vi "main.vi"() -> ()   [LabVIEW 2023] (continued)
 0CF102A7   00000004    8        30\t75\tE0\t2E\t80\tFF\tFF\tFD\r\n       463  0CF101A7   00000004    8        68\t00\t97\tCC\t00\t15\t39\t31\r\n       512  1FFFFFFF   00000004    8        00\t20\tFF\tFF\tFF\tFF\tFF\tFF\r\n       503  0CF102A7   00000004    8        30\t75\tE0\t2E\t80\tFF\tFF\tFD\r\n       503  0CF101A7   00000004    8        68\t00\t97\tCC\t00\t15\t39\t33\r\n       502  1FFFFFFF   00000004    8        00\t20\tFF\tFF\tFF\tFF\tFF\tFF\r\n       493  18F106A7   00000004    8        00\tF7\tFF\tFF\tFF\tFF\tFF\t7A\r\n       492  1FFFFFFF   00000004    8        00\t00\tFF\tFF\tFF\tFF\tFF\tFF\r\n       483  0CF102A7   00000004    8        30\t75\tE0\t2E\t80\tFF\tFF\tFD\r\n       483  0CF101A7   00000004    8        68\t00\t97\tCC\t00\t15\t39\t32\r\n       482  1FFFFFFF   00000004    8        00\t20\tFF\tFF\tFF\tFF\tFF\tFF\r\n       472  1FFFFFFF   00000004    8        00\t20\tFF\tFF\tFF\tFF\tFF\tFF\r\n       463  0CF102A7   00000004    8        30\t75\tE0\t2E\t80\tFF\tFF\tFD\r\n       522  1FFFFFFF   00000004    8        00\t20\tFF\tFF\tFF\tFF\tFF\tFF\r\n       512  1FFFFFFF   00000004    8        00\t20\tFF\tFF\tFF\tFF\tFF\tFF\r\n       503  0CF102A7   00000004    8        30\t75\tE0\t2E\t80\tFF\tFF\tFD\r\n       503  0CF101A7   00000004    8        68\t00\t97\tCC\t00\t15\t39\t33\r\n       502  1FFFFFFF   00000004    8        00\t20\tFF\tFF\tFF\tFF\tFF\tFF\r\n       493  18F106A7   00000004    8        00\tF7\tFF\tFF\tFF\tFF\tFF\t7A\r\n       492  1FFFFFFF   00000004    8        00\t00\tFF\tFF\tFF\tFF\tFF\tFF\r\n       483  0CF102A7   00000004    8        30\t75\tE0\t2E\t80\tFF\tFF\tFD\r\n       483  0CF101A7   00000004    8        68\t00\t97\tCC\t00\t15\t39\t32\r\n       482  1FFFFFFF   00000004    8        00\t20\tFF\tFF\tFF\tFF\tFF\tFF\r\n       472  1FFFFFFF   00000004    8        00\t20\tFF\tFF\tFF\tFF\tFF\tFF\r\n       523  0CF101A7   00000004    8        68\t00\t97\tCC\t00\t15\t39\t34\r\n       522  1FFFFFFF   00000004    8        00\t20\tFF\tFF\tFF\tFF\tFF\tFF\r\n       512  1FFFFFFF   00000004    8        00\t20\tFF\tFF\tFF\tFF\tFF\tFF\r\n       503  0CF102A7   00000004    8        30\t75\tE0\t2E\t80\tFF\tFF\tFD\r\n       503  0CF101A7   00000004    8        68\t00\t97\tCC\t00\t15\t39\t33\r\n       502  1FFFFFFF   00000004    8        00\t20\tFF\tFF\tFF\tFF\tFF\tFF\r\n       493  18F106A7   00000004    8        00\tF7\tFF\tFF\tFF\tFF\tFF\t7A\r\n       492  1FFFFFFF   00000004    8        00\t00\tFF\tFF\tFF\tFF\tFF\tFF\r\n       483  0CF102A7   00000004    8        30\t75\tE0\t2E\t80\tFF\tFF\tFD\r\n       483  0CF101A7   00000004    8        68\t00\t97\tCC\t00\t15\t39\t32\r\n       482  1FFFFFFF   00000004    8        00\t20\tFF\tFF\tFF\tFF\tFF\tFF\r\n       523  0CF102A7   00000004    8        30\t75\tE0\t2E\t80\tFF\tFF\tFD\r\n       523  0CF101A7   00000004    8        68\t00\t97\tCC\t00\t15\t39\t34\r\n       522  1FFFFFFF   00000004    8        00\t20\tFF\tFF\tFF\tFF\tFF\tFF\r\n       512  1FFFFFFF   00000004    8        00\t20\tFF\tFF\tFF\tFF\tFF\tFF\r\n       503  0CF102A7   00000004    8        30\t75\tE0\t2E\t80\tFF\tFF\tFD\r\n       503  0CF101A7   00000004    8        68\t00\t97\tCC\t00\t15\t39\t33\r\n       502  1FFFFFFF   00000004    8        00\t20\tFF\tFF\tFF\tFF\tFF\tFF\r\n       493  18F106A7   00000004    8        00\tF7\tFF\tFF\tFF\tFF\tFF\t7A\r\n       492  1FFFFFFF   00000004    8        00\t00\tFF\tFF\tFF\tFF\tFF\tFF\r\n       483  0CF102A7   00000004    8        30\t75\tE0\t2E\t80\tFF\tFF\tFD\r\n       483  0CF101A7   00000004    8        68\t00\t97\tCC\t00\t15\t39\t32\r\n       532  1FFFFFFF   00000004    8        00\t20\tFF\tFF\tFF\tFF\tFF\tFF\r\n       523  0CF102A7   00000004    8        30\t75\tE0\t2E\t80\tFF\tFF\tFD\r\n       523  0CF101A7   00000004    8        68\t00\t97\tCC\t00\t15\t39\t34\r\n       522  1FFFFFFF   00000004    8        00\t20\tFF\tFF\tFF\tFF\tFF\tFF\r\n       512  1FFFFFFF   00000004    8        00\t20\tFF\tFF\tFF\tFF\tFF\tFF\r\n       503  0CF102A7   00000004    8        30\t75\tE0\t2E\t80\tFF\tFF\tFD\r\n       503  0CF101A7   00000004    8        68\t00\t97\tCC\t00\t15\t39\t33\r\n       502  1FFFFFFF   00000004    8        00\t20\tFF\tFF\tFF\tFF\tFF\tFF\r\n       493  18F106A7   00000004    8        00\tF7\tFF\tFF\tFF\tFF\tFF\t7A\r\n       492  1FFFFFFF   00000004    8        00\t00\tFF\tFF\tFF\tFF\tFF\tFF\r\n       483  0CF102A7   00000004    8        30\t75\tE0\t2E\t80\tFF\tFF\tFD\r\n       541  18F11FF0   00000004    8        FF\t3F\t90\t68\t88\t1B\t10\tDC\r\n       532  1FFFFFFF   00000004    8        00\t20\tFF\tFF\tFF\tFF\tFF\tFF\r\n       523  0CF102A7   00000004    8        30\t75\tE0\t2E\t80\tFF\tFF\tFD\r\n       523  0CF101A7   00000004    8        68\t00\t97\tCC\t00\t15\t39\t34\r\n       522  1FFFFFFF   00000004    8        00\t20\tFF\tFF\tFF\tFF\tFF\tFF\r\n       512  1FFFFFFF   00000004    8        00\t20\tFF\tFF\tFF\tFF\tFF\tFF\r\n       503  0CF102A7   00000004    8        30\t75\tE0\t2E\t80\tFF\tFF\tFD\r\n       503  0CF101A7   00000004    8        68\t00\t97\tCC\t00\t15\t39\t33\r\n       502  1FFFFFFF   00000004    8        00\t20\tFF\tFF\tFF\tFF\tFF\tFF\r\n       493  18F106A7   00000004    8        00\tF7\tFF\tFF\tFF\tFF\tFF\t7A\r\n       492  1FFFFFFF   00000004    8        00\t00\tFF\tFF\tFF\tFF\tFF\tFF\r\n       542  18F120F0   00000004    8        2B\t75\t60\tB1\tB0\t01\tFF\tFF\r\n       541  18F11FF0   00000004    8        FF\t3F\t90\t68\t88\t1B\t10\tDC\r\n       532  1FFFFFFF   00000004    8        00\t20\tFF\tFF\tFF\tFF\tFF\tFF\r\n       523  0CF102A7   00000004    8        30\t75\tE0\t2E\t80\tFF\tFF\tFD\r\n       523  0CF101A7   00000004    8        68\t00\t97\tCC\t00\t15\t39\t34\r\n       522  1FFFFFFF   00000004    8        00\t20\tFF\tFF\tFF\tFF\tFF\tFF\r\n       512  1FFFFFFF   00000004    8        00\t20\tFF\tFF\tFF\tFF\tFF\tFF\r\n       503  0CF102A7   00000004    8        30\t75\tE0\t2E\t80\tFF\tFF\tFD\r\n       503  0CF101A7   00000004    8        68\t00\t97\tCC\t00\t15\t39\t33\r\n       502  1FFFFFFF   00000004    8        00\t20\tFF\tFF\tFF\tFF\tFF\tFF\r\n       493  18F106A7   00000004    8        00\tF7\tFF\tFF\tFF\tFF\tFF\t7A\r\n       543  0CF101A7   00000004    8        68\t00\t97\tCC\t00\t15\t39\t35\r\n       542  18F120F0   00000004    8        2B\t75\t60\tB1\tB0\t01\tFF\tFF\r\n       541  18F11FF0   00000004    8        FF\t3F\t90\t68\t88\t1B\t10\tDC\r\n       532  1FFFFFFF   00000004    8        00\t20\tFF\tFF\tFF\tFF\tFF\tFF\r\n       523  0CF102A7   00000004    8        30\t75\tE0\t2E\t80\tFF\tFF\tFD\r\n       523  0CF101A7   00000004    8        68\t00\t97\tCC\t00\t15\t39\t34\r\n       522  1FFFFFFF   00000004    8        00\t20\tFF\tFF\tFF\tFF\tFF\tFF\r\n       512  1FFFFFFF   00000004    8        00\t20\tFF\tFF\tFF\tFF\tFF\tFF\r\n       503  0CF102A7   00000004    8        30\t75\tE0\t2E\t80\tFF\tFF\tFD\r\n       503  0CF101A7   00000004    8        68\t00\t97\tCC\t00\t15\t39\t33\r\n       502  1FFFFFFF   00000004    8        00\t20\tFF\tFF\tFF\tFF\tFF\tFF\r\n       543  0C3C4D4A   00000004    8        BE\tFF\tFF\t7F\t18\tFF\tFF\t3D\r\n       543  0CF101A7   00000004    8        68\t00\t97\tCC\t00\t15\t39\t35\r\n       542  18F120F0   00000004    8        2B\t75\t60\tB1\tB0\t01\tFF\tFF\r\n       541  18F11FF0   00000004    8        FF\t3F\t90\t68\t88\t1B\t10\tDC\r\n       532  1FFFFFFF   00000004    8        00\t20\tFF\tFF\tFF\tFF\tFF\tFF\r\n       523  0CF102A7   00000004    8        30\t75\tE0\t2E\t80\tFF\tFF\tFD\r\n       523  0CF101A7   00000004    8        68\t00\t97\tCC\t00\t15\t39\t34\r\n       522  1FFFFFFF   00000004    8        00\t20\tFF\tFF\tFF\tFF\tFF\tFF\r\n       512  1FFFFFFF   00000004    8        00\t20\tFF\tFF\tFF\tFF\tFF\tFF\r\n       503  0CF102A7   00000004    8        30\t75\tE0\t2E\t80\tFF\tFF\tFD\r\n       503  0CF101A7   00000004    8        68\t00\t97\tCC\t00\t15\t39\t33\r\n       544  0CF102A7   00000004    8        30\t75\tE0\t2E\t80\tFF\tFF\tFD\r\n       543  0C3C4D4A   00000004    8        BE\tFF\tFF\t7F\t18\tFF\tFF\t3D\r\n       543  0CF101A7   00000004    8        68\t00\t97\tCC\t00\t15\t39\t35\r\n       542  18F120F0   00000004    8        2B\t75\t60\tB1\tB0\t01\tFF\tFF\r\n       541  18F11FF0   00000004    8        FF\t3F\t90\t68\t88\t1B\t10\tDC\r\n       532  1FFFFFFF   00000004    8        00\t20\tFF\tFF\tFF\tFF\tFF\tFF\r\n       523  0CF102A7   00000004    8        30\t75\tE0\t2E\t80\tFF\tFF\tFD\r\n       523  0CF101A7   00000004    8        68\t00\t97\tCC\t00\t15\t39\t34\r\n       522  1FFFFFFF   00000004    8        00\t20\tFF\tFF\tFF\tFF\tFF\tFF\r\n       512  1FFFFFFF   00000004    8        00\t20\tFF\tFF\tFF\tFF\tFF\tFF\r\n       503  0CF102A7   00000004    8        30\t75\tE0\t2E\t80\tFF\tFF\tFD\r\n       544  0CF103A7   00000004    8        17\t1F\t08\t60\tB1\t1F\t08\t3D\r\n       544  0CF102A7   00000004    8        30\t75\tE0\t2E\t80\tFF\tFF\tFD\r\n       543  0C3C4D4A   00000004    8        BE\tFF\tFF\t7F\t18\tFF\tFF\t3D\r\n       543  0CF101A7   00000004    8        68\t00\t97\tCC\t00\t15\t39\t35\r\n       542  18F120F0   00000004    8        2B\t75\t60\tB1\tB0\t01\tFF\tFF\r\n       541  18F11FF0   00000004    8        FF\t3F\t90\t68\t88\t1B\t10\tDC\r\n       532  1FFFFFFF   00000004    8        00\t20\tFF\tFF\tFF\tFF\tFF\tFF\r\n       523  0CF102A7   00000004    8        30\t75\tE0\t2E\t80\tFF\tFF\tFD\r\n       523  0CF101A7   00000004    8        68\t00\t97\tCC\t00\t15\t39\t34\r\n       522  1FFFFFFF   00000004    8        00\t20\tFF\tFF\tFF\tFF\tFF\tFF\r\n       512  1FFFFFFF   00000004    8        00\t20\tFF\tFF\tFF\tFF\tFF\tFF\r\n       545  0CF104A7   00000004    8        F0\t60\t22\tFC\tFF\tFF\tFF\t3D\r\n       544  0CF103A7   00000004    8        17\t1F\t08\t60\tB1\t1F\t08\t3D\r\n       544  0CF102A7   00000004    8        30\t75\tE0\t2E\t80\tFF\tFF\tFD\r\n       543  0C3C4D4A   00000004    8        BE\tFF\tFF\t7F\t18\tFF\tFF\t3D\r\n       543  0CF101A7   00000004    8        68\t00\t97\tCC\t00\t15\t39\t35\r\n       542  18F120F0   00000004    8        2B\t75\t60\tB1\tB0\t01\tFF\tFF\r\n       541  18F11FF0   00000004    8        FF\t3F\t90\t68\t88\t1B\t10\tDC\r\n       532  1FFFFFFF   00000004    8        00\t20\tFF\tFF\tFF\tFF\tFF\tFF\r\n       523  0CF102A7   00000004    8        30\t75\tE0\t2E\t80\tFF\tFF\tFD\r\n       523  0CF101A7   00000004    8        68\t00\t97\tCC\t00\t15\t39\t34\r\n       522  1FFFFFFF   00000004    8        00\t20\tFF\tFF\tFF\tFF\tFF\tFF\r\n       545  18F106A7   00000004    8        00\tF7\tFF\tFF\tFF\tFF\tFF\t7B\r\n       545  0CF104A7   00000004    8        F0\t60\t22\tFC\tFF\tFF\tFF\t3D\r\n       544  0CF103A7   00000004    8        17\t1F\t08\t60\tB1\t1F\t08\t3D\r\n       544  0CF102A7   00000004    8        30\t75\tE0\t2E\t80\tFF\tFF\tFD\r\n       543  0C3C4D4A   00000004    8        BE\tFF\tFF\t7F\t18\tFF\tFF\t3D\r\n       543  0CF101A7   00000004    8        68\t00\t97\tCC\t00\t15\t39\t35\r\n       542  18F120F0   00000004    8        2B\t75\t60\tB1\tB0\t01\tFF\tFF\r\n       541  18F11FF0   00000004    8        FF\t3F\t90\t68\t88\t1B\t10\tDC\r\n       532  1FFFFFFF   00000004    8        00\t20\tFF\tFF\tFF\tFF\tFF\tFF\r\n       523  0CF102A7   00000004    8        30\t75\tE0\t2E\t80\tFF\tFF\tFD\r\n       523  0CF101A7   00000004    8        68\t00\t97\tCC\t00\t15\t39\t34\r\n       546  18F121F0   00000004    8        09\t16\t00\t00\tFF\tFF\tB0\t01\r\n       545  18F106A7   00000004    8        00\tF7\tFF\tFF\tFF\tFF\tFF\t7B\r\n       545  0CF104A7   00000004    8        F0\t60\t22\tFC\tFF\tFF\tFF\t3D\r\n       544  0CF103A7   00000004    8        17\t1F\t08\t60\tB1\t1F\t08\t3D\r\n       544  0CF102A7   00000004    8        30\t75\tE0\t2E\t80\tFF\tFF\tFD\r\n       543  0C3C4D4A   00000004    8        BE\tFF\tFF\t7F\t18\tFF\tFF\t3D\r\n       543  0CF101A7   00000004    8        68\t00\t97\tCC\t00\t15\t39\t35\r\n       542  18F120F0   00000004    8        2B\t75\t60\tB1\tB0\t01\tFF\tFF\r\n       541  18F11FF0   00000004    8        FF\t3F\t90\t68\t88\t1B\t10\tDC\r\n       532  1FFFFFFF   00000004    8        00\t20\tFF\tFF\tFF\tFF\tFF\tFF\r\n       523  0CF102A7   00000004    8        30\t75\tE0\t2E\t80\tFF\tFF\tFD\r\n       547  1FFFFFFF   00000004    8        00\t00\tFF\tFF\tFF\tFF\tFF\tFF\r\n       546  18F121F0   00000004    8        09\t16\t00\t00\tFF\tFF\tB0\t01\r\n       545  18F106A7   00000004    8        00\tF7\tFF\tFF\tFF\tFF\tFF\t7B\r\n       545  0CF104A7   00000004    8        F0\t60\t22\tFC\tFF\tFF\tFF\t3D\r\n       544  0CF103A7   00000004    8        17\t1F\t08\t60\tB1\t1F\t08\t3D\r\n       544  0CF102A7   00000004    8        30\t75\tE0\t2E\t80\tFF\tFF\tFD\r\n       543  0C3C4D4A   00000004    8        BE\tFF\tFF\t7F\t18\tFF\tFF\t3D\r\n       543  0CF101A7   00000004    8        68\t00\t97\tCC\t00\t15\t39\t35\r\n       542  18F120F0   00000004    8        2B\t75\t60\tB1\tB0\t01\tFF\tFF\r\n       541  18F11FF0   00000004    8        FF\t3F\t90\t68\t88\t1B\t10\tDC\r\n       532  1FFFFFFF   00000004    8        00\t20\tFF\tFF\tFF\tFF\tFF\tFF\r\n       552  1FFFFFFF   00000004    8        00\t20\tFF\tFF\tFF\tFF\tFF\tFF\r\n       547  1FFFFFFF   00000004    8        00\t00\tFF\tFF\tFF\tFF\tFF\tFF\r\n       546  18F121F0   00000004    8        09\t16\t00\t00\tFF\tFF\tB0\t01\r\n       545  18F106A7   00000004    8        00\tF7\tFF\tFF\tFF\tFF\tFF\t7B\r\n       545  0CF104A7   00000004    8        F0\t60\t22\tFC\tFF\tFF\tFF\t3D\r\n       544  0CF103A7   00000004    8        17\t1F\t08\t60\tB1\t1F\t08\t3D\r\n       544  0CF102A7   00000004    8        30\t75\tE0\t2E\t80\tFF\tFF\tFD\r\n       543  0C3C4D4A   00000004    8        BE\tFF\tFF\t7F\t18\tFF\tFF\t3D\r\n       543  0CF101A7   00000004    8        68\t00\t97\tCC\t00\t15\t39\t35\r\n       542  18F120F0   00000004    8        2B\t75\t60\tB1\tB0\t01\tFF\tFF\r\n       541  18F11FF0   00000004    8        FF\t3F\t90\t68\t88\t1B\t10\tDC\r\n       562  1FFFFFFF   00000004    8        00\t00\tFF\tFF\tFF\tFF\tFF\tFF\r\n       552  1FFFFFFF   00000004    8        00\t20\tFF\tFF\tFF\tFF\tFF\tFF\r\n       547  1FFFFFFF   00000004    8        00\t00\tFF\tFF\tFF\tFF\tFF\tFF\r\n       546  18F121F0   00000004    8        09\t16\t00\t00\tFF\tFF\tB0\t01\r\n       545  18F106A7   00000004    8        00\tF7\tFF\tFF\tFF\tFF\tFF\t7B\r\n       545  0CF104A7   00000004    8        F0\t60\t22\tFC\tFF\tFF\tFF\t3D\r\n       544  0CF103A7   00000004    8        17\t1F\t08\t60\tB1\t1F\t08\t3D\r\n       544  0CF102A7   00000004    8        30\t75\tE0\t2E\t80\tFF\tFF\tFD\r\n       543  0C3C4D4A   00000004    8        BE\tFF\tFF\t7F\t18\tFF\tFF\t3D\r\n       543  0CF101A7   00000004    8        68\t00\t97\tCC\t00\t15\t39\t35\r\n       542  18F120F0   00000004    8        2B\t75\t60\tB1\tB0\t01\tFF\tFF\r\n       563  0CF101A7   00000004    8        68\t00\t97\tCC\t00\t15\t39\t36\r\n       562  1FFFFFFF   00000004    8        00\t00\tFF\tFF\tFF\tFF\tFF\tFF\r\n       552  1FFFFFFF   00000004    8        00\t20\tFF\tFF\tFF\tFF\tFF\tFF\r\n       547  1FFFFFFF   00000004    8        00\t00\tFF\tFF\tFF\tFF\tFF\tFF\r\n       546  18F121F0   00000004    8        09\t16\t00\t00\tFF\tFF\tB0\t01\r\n       545  18F106A7   00000004    8        00\tF7\tFF\tFF\tFF\tFF\tFF\t7B\r\n       545  0CF104A7   00000004    8        F0\t60\t22\tFC\tFF\tFF\tFF\t3D\r\n       544  0CF103A7   00000004    8        17\t1F\t08\t60\tB1\t1F\t08\t3D\r\n       544  0CF102A7   00000004    8        30\t75\tE0\t2E\t80\tFF\tFF\tFD\r\n       543  0C3C4D4A   00000004    8        BE\tFF\tFF\t7F\t18\tFF\tFF\t3D\r\n       543  0CF101A7   00000004    8        68\t00\t97\tCC\t00\t15\t39\t35\r\n       563  0CF102A7   00000004    8        30\t75\tE0\t2E\t80\tFF\tFF\tFD\r\n       563  0CF101A7   00000004    8        68\t00\t97\tCC\t00\t15\t39\t36\r\n       562  1FFFFFFF   00000004    8        00\t00\tFF\tFF\tFF\tFF\tFF\tFF\r\n       552  1FFFFFFF   00000004    8        00\t20\tFF\tFF\tFF\tFF\tFF\tFF\r\n       547  1FFFFFFF   00000004    8        00\t00\tFF\tFF\tFF\tFF\tFF\tFF\r\n       546  18F121F0   00000004    8        09\t16\t00\t00\tFF\tFF\tB0\t01\r\n       545  18F106A7   00000004    8        00\tF7\tFF\tFF\tFF\tFF\tFF\t7B\r\n       545  0CF104A7   00000004    8        F0\t60\t22\tFC\tFF\tFF\tFF\t3D\r\n       544  0CF103A7   00000004    8        17\t1F\t08\t60\tB1\t1F\t08\t3D\r\n       544  0CF102A7   00000004    8        30\t75\tE0\t2E\t80\tFF\tFF\tFD\r\n       543  0C3C4D4A   00000004    8        BE\tFF\tFF\t7F\t18\tFF\tFF\t3D\r\n       572  1FFFFFFF   00000004    8        00\t20\tFF\tFF\tFF\tFF\tFF\tFF\r\n       563  0CF102A7   00000004    8        30\t75\tE0\t2E\t80\tFF\tFF\tFD\r\n       563  0CF101A7   00000004    8        68\t00\t97\tCC\t00\t15\t39\t36\r\n       562  1FFFFFFF   00000004    8        00\t00\tFF\tFF\tFF\tFF\tFF\tFF\r\n       552  1FFFFFFF   00000004    8        00\t20\tFF\tFF\tFF\tFF\tFF\tFF\r\n       547  1FFFFFFF   00000004    8        00\t00\tFF\tFF\tFF\tFF\tFF\tFF\r\n       546  18F121F0   00000004    8        09\t16\t00\t00\tFF\tFF\tB0\t01\r\n       545  18F106A7   00000004    8        00\tF7\tFF\tFF\tFF\tFF\tFF\t7B\r\n       545  0CF104A7   00000004    8        F0\t60\t22\tFC\tFF\tFF\tFF\t3D\r\n       544  0CF103A7   00000004    8        17\t1F\t08\t60\tB1\t1F\t08\t3D\r\n       544  0CF102A7   00000004    8        30\t75\tE0\t2E\t80\tFF\tFF\tFD\r\n       582  1FFFFFFF   00000004    8        00\t20\tFF\tFF\tFF\tFF\tFF\tFF\r\n       572  1FFFFFFF   00000004    8        00\t20\tFF\tFF\tFF\tFF\tFF\tFF\r\n       563  0CF102A7   00000004    8        30\t75\tE0\t2E\t80\tFF\tFF\tFD\r\n       563  0CF101A7   00000004    8        68\t00\t97\tCC\t00\t15\t39\t36\r\n       562  1FFFFFFF   00000004    8        00\t00\tFF\tFF\tFF\tFF\tFF\tFF\r\n       552  1FFFFFFF   00000004    8        00\t20\tFF\tFF\tFF\tFF\tFF\tFF\r\n       547  1FFFFFFF   00000004    8        00\t00\tFF\tFF\tFF\tFF\tFF\tFF\r\n       546  18F121F0   00000004    8        09\t16\t00\t00\tFF\tFF\tB0\t01\r\n       545  18F106A7   00000004    8        00\tF7\tFF\tFF\tFF\tFF\tFF\t7B\r\n       545  0CF104A7   00000004    8        F0\t60\t22\tFC\tFF\tFF\tFF\t3D\r\n       544  0CF103A7   00000004    8        17\t1F\t08\t60\tB1\t1F\t08\t3D\r\n       583  0CF101A7   00000004    8        68\t00\t97\tCC\t00\t15\t39\t37\r\n       582  1FFFFFFF   00000004    8        00\t20\tFF\tFF\tFF\tFF\tFF\tFF\r\n       572  1FFFFFFF   00000004    8        00\t20\tFF\tFF\tFF\tFF\tFF\tFF\r\n       563  0CF102A7   00000004    8        30\t75\tE0\t2E\t80\tFF\tFF\tFD\r\n       563  0CF101A7   00000004    8        68\t00\t97\tCC\t00\t15\t39\t36\r\n       562  1FFFFFFF   00000004    8        00\t00\tFF\tFF\tFF\tFF\tFF\tFF\r\n       552  1FFFFFFF   00000004    8        00\t20\tFF\tFF\tFF\tFF\tFF\tFF\r\n       547  1FFFFFFF   00000004    8        00\t00\tFF\tFF\tFF\tFF\tFF\tFF\r\n       546  18F121F0   00000004    8        09\t16\t00\t00\tFF\tFF\tB0\t01\r\n       545  18F106A7   00000004    8        00\tF7\tFF\tFF\tFF\tFF\tFF\t7B\r\n       545  0CF104A7   00000004    8        F0\t60\t22\tFC\tFF\tFF\tFF\t3D\r\n       583  0CF102A7   00000004    8        30\t75\tE0\t2E\t80\tFF\tFF\tFD\r\n       583  0CF101A7   00000004    8        68\t00\t97\tCC\t00\t15\t39\t37\r\n       582  1FFFFFFF   00000004    8        00\t20\tFF\tFF\tFF\tFF\tFF\tFF\r\n       572  1FFFFFFF   00000004    8        00\t20\tFF\tFF\tFF\tFF\tFF\tFF\r\n       563  0CF102A7   00000004    8        30\t75\tE0\t2E\t80\tFF\tFF\tFD\r\n       563  0CF101A7   00000004    8        68\t00\t97\tCC\t00\t15\t39\t36\r\n       562  1FFFFFFF   00000004    8        00\t00\tFF\tFF\tFF\tFF\tFF\tFF\r\n       552  1FFFFFFF   00000004    8        00\t20\tFF\tFF\tFF\tFF\tFF\tFF\r\n       547  1FFFFFFF   00000004    8        00\t00\tFF\tFF\tFF\tFF\tFF\tFF\r\n       546  18F121F0   00000004    8        09\t16\t00\t00\tFF\tFF\tB0\t01\r\n       545  18F106A7   00000004    8        00\tF7\tFF\tFF\tFF\tFF\tFF\t7B\r\n       592  1FFFFFFF   00000004    8        00\t00\tFF\tFF\tFF\tFF\tFF\tFF\r\n       583  0CF102A7   00000004    8        30\t75\tE0\t2E\t80\tFF\tFF\tFD\r\n       583  0CF101A7   00000004    8        68\t00\t97\tCC\t00\t15\t39\t37\r\n       582  1FFFFFFF   00000004    8        00\t20\tFF\tFF\tFF\tFF\tFF\tFF\r\n       572  1FFFFFFF   00000004    8        00\t20\tFF\tFF\tFF\tFF\tFF\tFF\r\n       563  0CF102A7   00000004    8        30\t75\tE0\t2E\t80\tFF\tFF\tFD\r\n       563  0CF101A7   00000004    8        68\t00\t97\tCC\t00\t15\t39\t36\r\n       562  1FFFFFFF   00000004    8        00\t00\tFF\tFF\tFF\tFF\tFF\tFF\r\n       552  1FFFFFFF   00000004    8        00\t20\tFF\tFF\tFF\tFF\tFF\tFF\r\n       547  1FFFFFFF   00000004    8        00\t00\tFF\tFF\tFF\tFF\tFF\tFF\r\n       546  18F121F0   00000004    8        09\t16\t00\t00\tFF\tFF\tB0\t01\r\n       593  18F106A7   00000004    8        00\tF7\tFF\tFF\tFF\tFF\tFF\t7C\r\n       592  1FFFFFFF   00000004    8        00\t00\tFF\tFF\tFF\tFF\tFF\tFF\r\n       583  0CF102A7   00000004    8        30\t75\tE0\t2E\t80\tFF\tFF\tFD\r\n       583  0CF101A7   00000004    8        68\t00\t97\tCC\t00\t15\t39\t37\r\n       582  1FFFFFFF   00000004    8        00\t20\tFF\tFF\tFF\tFF\tFF\tFF\r\n       572  1FFFFFFF   00000004    8        00\t20\tFF\tFF\tFF\tFF\tFF\tFF\r\n       563  0CF102A7   00000004    8        30\t75\tE0\t2E\t80\tFF\tFF\tFD\r\n       563  0CF101A7   00000004    8        68\t00\t97\tCC\t00\t15\t39\t36\r\n       562  1FFFFFFF   00000004    8        00\t00\tFF\tFF\tFF\tFF\tFF\tFF\r\n       552  1FFFFFFF   00000004    8        00\t20\tFF\tFF\tFF\tFF\tFF\tFF\r\n       547  1FFFFFFF   00000004    8        00\t00\tFF\tFF\tFF\tFF\tFF\tFF\r\n       602  1FFFFFFF   00000004    8        00\t20\tFF\tFF\tFF\tFF\tFF\tFF\r\n       593  18F106A7   00000004    8        00\tF7\tFF\tFF\tFF\tFF\tFF\t7C\r\n       592  1FFFFFFF   00000004    8        00\t00\tFF\tFF\tFF\tFF\tFF\tFF\r\n       583  0CF102A7   00000004    8        30\t75\tE0\t2E\t80\tFF\tFF\tFD\r\n       583  0CF101A7   00000004    8        68\t00\t97\tCC\t00\t15\t39\t37\r\n       582  1FFFFFFF   00000004    8        00\t20\tFF\tFF\tFF\tFF\tFF\tFF\r\n       572  1FFFFFFF   00000004    8        00\t20\tFF\tFF\tFF\tFF\tFF\tFF\r\n       563  0CF102A7   00000004    8        30\t75\tE0\t2E\t80\tFF\tFF\tFD\r\n       563  0CF101A7   00000004    8        68\t00\t97\tCC\t00\t15\t39\t36\r\n       562  1FFFFFFF   00000004    8        00\t00\tFF\tFF\tFF\tFF\tFF\tFF\r\n       552  1FFFFFFF   00000004    8        00\t20\tFF\tFF\tFF\tFF\tFF\tFF\r\n       603  0CF101A7   00000004    8        68\t00\t97\tCC\t00\t15\t39\t38\r\n       602  1FFFFFFF   00000004    8        00\t20\tFF\tFF\tFF\tFF\tFF\tFF\r\n       593  18F106A7   00000004    8        00\tF7\tFF\tFF\tFF\tFF\tFF\t7C\r\n       592  1FFFFFFF   00000004    8        00\t00\tFF\tFF\tFF\tFF\tFF\tFF\r\n       583  0CF102A7   00000004    8        30\t75\tE0\t2E\t80\tFF\tFF\tFD\r\n       583  0CF101A7   00000004    8        68\t00\t97\tCC\t00\t15\t39\t37\r\n       582  1FFFFFFF   00000004    8        00\t20\tFF\tFF\tFF\tFF\tFF\tFF\r\n       572  1FFFFFFF   00000004    8        00\t20\tFF\tFF\tFF\tFF\tFF\tFF\r\n       563  0CF102A7   00000004    8        30\t75\tE0\t2E\t80\tFF\tFF\tFD\r\n       563  0CF101A7   00000004    8        68\t00\t97\tCC\t00\t15\t39\t36\r\n       562  1FFFFFFF   00000004    8        00\t00\tFF\tFF\tFF\tFF\tFF\tFF\r\n       603  0CF102A7   00000004    8        30\t75\tE0\t2E\t80\tFF\tFF\tFD\r\n       603  0CF101A7   00000004    8        68\t00\t97\tCC\t00\t15\t39\t38\r\n       602  1FFFFFFF   00000004    8        00\t20\tFF\tFF\tFF\tFF\tFF\tFF\r\n       593  18F106A7   00000004    8        00\tF7\tFF\tFF\tFF\tFF\tFF\t7C\r\n       592  1FFFFFFF   00000004    8        00\t00\tFF\tFF\tFF\tFF\tFF\tFF\r\n       583  0CF102A7   00000004    8        30\t75\tE0\t2E\t80\tFF\tFF\tFD\r\n       583  0CF101A7   00000004    8        68\t00\t97\tCC\t00\t15\t39\t37\r\n       582  1FFFFFFF   00000004    8        00\t20\tFF\tFF\tFF\tFF\tFF\tFF\r\n       572  1FFFFFFF   00000004    8        00\t20\tFF\tFF\tFF\tFF\tFF\tFF\r\n       563  0CF102A7   00000004    8        30\t75\tE0\t2E\t80\tFF\tFF\tFD\r\n       563  0CF101A7   00000004    8        68\t00\t97\tCC\t00\t15\t39\t36\r\n       612  1FFFFFFF   00000004    8        00\t00\tFF\tFF\tFF\tFF\tFF\tFF\r\n       603  0CF102A7   00000004    8        30\t75\tE0\t2E\t80\tFF\tFF\tFD\r\n       603  0CF101A7   00000004    8        68\t00\t97\tCC\t00\t15\t39\t38\r\n       602  1FFFFFFF   00000004    8        00\t20\tFF\tFF\tFF\tFF\tFF\tFF\r\n       593  18F106A7   00000004    8        00\tF7\tFF\tFF\tFF\tFF\tFF\t7C\r\n       592  1FFFFFFF   00000004    8        00\t00\tFF\tFF\tFF\tFF\tFF\tFF\r\n       583  0CF102A7   00000004    8        30\t75\tE0\t2E\t80\tFF\tFF\tFD\r\n       583  0CF101A7   00000004    8        68\t00\t97\tCC\t00\t15\t39\t37\r\n       582  1FFFFFFF   00000004    8        00\t20\tFF\tFF\tFF\tFF\tFF\tFF\r\n       572  1FFFFFFF   00000004    8        00\t20\tFF\tFF\tFF\tFF\tFF\tFF\r\n       563  0CF102A7   00000004    8        30\t75\tE0\t2E\t80\tFF\tFF\tFD\r\n       622  1FFFFFFF   00000004    8        00\t00\tFF\tFF\tFF\tFF\tFF\tFF\r\n       612  1FFFFFFF   00000004    8        00\t00\tFF\tFF\tFF\tFF\tFF\tFF\r\n       603  0CF102A7   00000004    8        30\t75\tE0\t2E\t80\tFF\tFF\tFD\r\n       603  0CF101A7   00000004    8        68\t00\t97\tCC\t00\t15\t39\t38\r\n       602  1FFFFFFF   00000004    8        00\t20\tFF\tFF\tFF\tFF\tFF\tFF\r\n       593  18F106A7   00000004    8        00\tF7\tFF\tFF\tFF\tFF\tFF\t7C\r\n       592  1FFFFFFF   00000004    8        00\t00\tFF\tFF\tFF\tFF\tFF\tFF\r\n       583  0CF102A7   00000004    8        30\t75\tE0\t2E\t80\tFF\tFF\tFD\r\n       583  0CF101A7   00000004    8        68\t00\t97\tCC\t00\t15\t39\t37\r\n       582  1FFFFFFF   00000004    8        00\t20\tFF\tFF\tFF\tFF\tFF\tFF\r\n       572  1FFFFFFF   00000004    8        00\t20\tFF\tFF\tFF\tFF\tFF\tFF\r\n       623  0CF101A7   00000004    8        68\t00\t97\tCC\t00\t15\t39\t39\r\n       622  1FFFFFFF   00000004    8        00\t00\tFF\tFF\tFF\tFF\tFF\tFF\r\n       612  1FFFFFFF   00000004    8        00\t00\tFF\tFF\tFF\tFF\tFF\tFF\r\n       603  0CF102A7   00000004    8        30\t75\tE0\t2E\t80\tFF\tFF\tFD\r\n       603  0CF101A7   00000004    8        68\t00\t97\tCC\t00\t15\t39\t38\r\n       602  1FFFFFFF   00000004    8        00\t20\tFF\tFF\tFF\tFF\tFF\tFF\r\n       593  18F106A7   00000004    8        00\tF7\tFF\tFF\tFF\tFF\tFF\t7C\r\n       592  1FFFFFFF   00000004    8        00\t00\tFF\tFF\tFF\tFF\tFF\tFF\r\n       583  0CF102A7   00000004    8        30\t75\tE0\t2E\t80\tFF\tFF\tFD\r\n       583  0CF101A7   00000004    8        68\t00\t97\tCC\t00\t15\t39\t37\r\n       582  1FFFFFFF   00000004    8        00\t20\tFF\tFF\tFF\tFF\tFF\tFF\r\n       623  0CF102A7   00000004    8        30\t75\tE0\t2E\t80\tFF\tFF\tFD\r\n       623  0CF101A7   00000004    8        68\t00\t97\tCC\t00\t15\t39\t39\r\n       622  1FFFFFFF   00000004    8        00\t00\tFF\tFF\tFF\tFF\tFF\tFF\r\n       612  1FFFFFFF   00000004    8        00\t00\tFF\tFF\tFF\tFF\tFF\tFF\r\n       603  0CF102A7   00000004    8        30\t75\tE0\t2E\t80\tFF\tFF\tFD\r\n       603  0CF101A7   00000004    8        68\t00\t97\tCC\t00\t15\t39\t38\r\n       602  1FFFFFFF   00000004    8        00\t20\tFF\tFF\tFF\tFF\tFF\tFF\r\n       593  18F106A7   00000004    8        00\tF7\tFF\tFF\tFF\tFF\tFF\t7C\r\n       592  1FFFFFFF   00000004    8        00\t00\tFF\tFF\tFF\tFF\tFF\tFF\r\n       583  0CF102A7   00000004    8        30\t75\tE0\t2E\t80\tFF\tFF\tFD\r\n       583  0CF101A7   00000004    8        68\t00\t97\tCC\t00\t15\t39\t37\r\n       632  1FFFFFFF   00000004    8        00\t20\tFF\tFF\tFF\tFF\tFF\tFF\r\n       623  0CF102A7   00000004    8        30\t75\tE0\t2E\t80\tFF\tFF\tFD\r\n       623  0CF101A7   00000004    8        68\t00\t97\tCC\t00\t15\t39\t39\r\n       622  1FFFFFFF   00000004    8        00\t00\tFF\tFF\tFF\tFF\tFF\tFF\r\n       612  1FFFFFFF   00000004    8        00\t00\tFF\tFF\tFF\tFF\tFF\tFF\r\n       603  0CF102A7   00000004    8        30\t75\tE0\t2E\t80\tFF\tFF\tFD\r\n       603  0CF101A7   00000004    8        68\t00\t97\tCC\t00\t15\t39\t38\r\n       602  1FFFFFFF   00000004    8        00\t20\tFF\tFF\tFF\tFF\tFF\tFF\r\n       593  18F106A7   00000004    8        00\tF7\tFF\tFF\tFF\tFF\tFF\t7C\r\n       592  1FFFFFFF   00000004    8        00\t00\tFF\tFF\tFF\tFF\tFF\tFF\r\n       583  0CF102A7   00000004    8        30\t75\tE0\t2E\t80\tFF\tFF\tFD\r\n       642  18F11FF0   00000004    8        FF\t3F\t90\t68\t88\t1B\t10\tEC\r\n       632  1FFFFFFF   00000004    8        00\t20\tFF\tFF\tFF\tFF\tFF\tFF\r\n       623  0CF102A7   00000004    8        30\t75\tE0\t2E\t80\tFF\tFF\tFD\r\n       623  0CF101A7   00000004    8        68\t00\t97\tCC\t00\t15\t39\t39\r\n       622  1FFFFFFF   00000004    8        00\t00\tFF\tFF\tFF\tFF\tFF\tFF\r\n       612  1FFFFFFF   00000004    8        00\t00\tFF\tFF\tFF\tFF\tFF\tFF\r\n       603  0CF102A7   00000004    8        30\t75\tE0\t2E\t80\tFF\tFF\tFD\r\n       603  0CF101A7   00000004    8        68\t00\t97\tCC\t00\t15\t39\t38\r\n       602  1FFFFFFF   00000004    8        00\t20\tFF\tFF\tFF\tFF\tFF\tFF\r\n       593  18F106A7   00000004    8        00\tF7\tFF\tFF\tFF\tFF\tFF\t7C\r\n       592  1FFFFFFF   00000004    8        00\t00\tFF\tFF\tFF\tFF\tFF\tFF\r\n       643  0CF101A7   00000004    8        68\t00\t97\tCC\t00\t15\t39\t3A\r\n       642  18F11FF0   00000004    8        FF\t3F\t90\t68\t88\t1B\t10\tEC\r\n       632  1FFFFFFF   00000004    8        00\t20\tFF\tFF\tFF\tFF\tFF\tFF\r\n       623  0CF102A7   00000004    8        30\t75\tE0\t2E\t80\tFF\tFF\tFD\r\n       623  0CF101A7   00000004    8        68\t00\t97\tCC\t00\t15\t39\t39\r\n       622  1FFFFFFF   00000004    8        00\t00\tFF\tFF\tFF\tFF\tFF\tFF\r\n       612  1FFFFFFF   00000004    8        00\t00\tFF\tFF\tFF\tFF\tFF\tFF\r\n       603  0CF102A7   00000004    8        30\t75\tE0\t2E\t80\tFF\tFF\tFD\r\n       603  0CF101A7   00000004    8        68\t00\t97\tCC\t00\t15\t39\t38\r\n       602  1FFFFFFF   00000004    8        00\t20\tFF\tFF\tFF\tFF\tFF\tFF\r\n       593  18F106A7   00000004    8        00\tF7\tFF\tFF\tFF\tFF\tFF\t7C\r\n       643  0CF102A7   00000004    8        30\t75\tE0\t2E\t80\tFF\tFF\tFD\r\n       643  0CF101A7   00000004    8        68\t00\t97\tCC\t00\t15\t39\t3A\r\n       642  18F11FF0   00000004    8        FF\t3F\t90\t68\t88\t1B\t10\tEC\r\n       632  1FFFFFFF   00000004    8        00\t20\tFF\tFF\tFF\tFF\tFF\tFF\r\n       623  0CF102A7   00000004    8        30\t75\tE0\t2E\t80\tFF\tFF\tFD\r\n       623  0CF101A7   00000004    8        68\t00\t97\tCC\t00\t15\t39\t39\r\n       622  1FFFFFFF   00000004    8        00\t00\tFF\tFF\tFF\tFF\tFF\tFF\r\n       612  1FFFFFFF   00000004    8        00\t00\tFF\tFF\tFF\tFF\tFF\tFF\r\n       603  0CF102A7   00000004    8        30\t75\tE0\t2E\t80\tFF\tFF\tFD\r\n       603  0CF101A7   00000004    8        68\t00\t97\tCC\t00\t15\t39\t38\r\n       602  1FFFFFFF   00000004    8        00\t20\tFF\tFF\tFF\tFF\tFF\tFF\r\n       644  0C3C4D4A   00000004    8        BE\tFF\tFF\t7F\t18\tFF\tFF\t3E\r\n       643  0CF102A7   00000004    8        30\t75\tE0\t2E\t80\tFF\tFF\tFD\r\n       643  0CF101A7   00000004    8        68\t00\t97\tCC\t00\t15\t39\t3A\r\n       642  18F11FF0   00000004    8        FF\t3F\t90\t68\t88\t1B\t10\tEC\r\n       632  1FFFFFFF   00000004    8        00\t20\tFF\tFF\tFF\tFF\tFF\tFF\r\n       623  0CF102A7   00000004    8        30\t75\tE0\t2E\t80\tFF\tFF\tFD\r\n       623  0CF101A7   00000004    8        68\t00\t97\tCC\t00\t15\t39\t39\r\n       622  1FFFFFFF   00000004    8        00\t00\tFF\tFF\tFF\tFF\tFF\tFF\r\n       612  1FFFFFFF   00000004    8        00\t00\tFF\tFF\tFF\tFF\tFF\tFF\r\n       603  0CF102A7   00000004    8        30\t75\tE0\t2E\t80\tFF\tFF\tFD\r\n       603  0CF101A7   00000004    8        68\t00\t97\tCC\t00\t15\t39\t38\r\n       644  0CF103A7   00000004    8        17\t1F\t08\t60\tB1\t1F\t08\t3E\r\n       644  0C3C4D4A   00000004    8        BE\tFF\tFF\t7F\t18\tFF\tFF\t3E\r\n       643  0CF102A7   00000004    8        30\t75\tE0\t2E\t80\tFF\tFF\tFD\r\n       643  0CF101A7   00000004    8        68\t00\t97\tCC\t00\t15\t39\t3A\r\n       642  18F11FF0   00000004    8        FF\t3F\t90\t68\t88\t1B\t10\tEC\r\n       632  1FFFFFFF   00000004    8        00\t20\tFF\tFF\tFF\tFF\tFF\tFF\r\n       623  0CF102A7   00000004    8        30\t75\tE0\t2E\t80\tFF\tFF\tFD\r\n       623  0CF101A7   00000004    8        68\t00\t97\tCC\t00\t15\t39\t39\r\n       622  1FFFFFFF   00000004    8        00\t00\tFF\tFF\tFF\tFF\tFF\tFF\r\n       612  1FFFFFFF   00000004    8        00\t00\tFF\tFF\tFF\tFF\tFF\tFF\r\n       603  0CF102A7   00000004    8        30\t75\tE0\t2E\t80\tFF\tFF\tFD\r\n       645  0CF104A7   00000004    8        F0\t60\t22\tFC\tFF\tFF\tFF\t3E\r\n       644  0CF103A7   00000004    8        17\t1F\t08\t60\tB1\t1F\t08\t3E\r\n       644  0C3C4D4A   00000004    8        BE\tFF\tFF\t7F\t18\tFF\tFF\t3E\r\n       643  0CF102A7   00000004    8        30\t75\tE0\t2E\t80\tFF\tFF\tFD\r\n       643  0CF101A7   00000004    8        68\t00\t97\tCC\t00\t15\t39\t3A\r\n       642  18F11FF0   00000004    8        FF\t3F\t90\t68\t88\t1B\t10\tEC\r\n       632  1FFFFFFF   00000004    8        00\t20\tFF\tFF\tFF\tFF\tFF\tFF\r\n       623  0CF102A7   00000004    8        30\t75\tE0\t2E\t80\tFF\tFF\tFD\r\n       623  0CF101A7   00000004    8        68\t00\t97\tCC\t00\t15\t39\t39\r\n       622  1FFFFFFF   00000004    8        00\t00\tFF\tFF\tFF\tFF\tFF\tFF\r\n       612  1FFFFFFF   00000004    8        00\t00\tFF\tFF\tFF\tFF\tFF\tFF\r\n       645  0CF105A7   00000004    8        94\t11\t00\t55\tFF\tFF\tFF\t1F\r\n       645  0CF104A7   00000004    8        F0\t60\t22\tFC\tFF\tFF\tFF\t3E\r\n       644  0CF103A7   00000004    8        17\t1F\t08\t60\tB1\t1F\t08\t3E\r\n       644  0C3C4D4A   00000004    8        BE\tFF\tFF\t7F\t18\tFF\tFF\t3E\r\n       643  0CF102A7   00000004    8        30\t75\tE0\t2E\t80\tFF\tFF\tFD\r\n       643  0CF101A7   00000004    8        68\t00\t97\tCC\t00\t15\t39\t3A\r\n       642  18F11FF0   00000004    8        FF\t3F\t90\t68\t88\t1B\t10\tEC\r\n       632  1FFFFFFF   00000004    8        00\t20\tFF\tFF\tFF\tFF\tFF\tFF\r\n       623  0CF102A7   00000004    8        30\t75\tE0\t2E\t80\tFF\tFF\tFD\r\n       623  0CF101A7   00000004    8        68\t00\t97\tCC\t00\t15\t39\t39\r\n       622  1FFFFFFF   00000004    8        00\t00\tFF\tFF\tFF\tFF\tFF\tFF\r\n       646  18F106A7   00000004    8        00\tF7\tFF\tFF\tFF\tFF\tFF\t7D\r\n       645  0CF105A7   00000004    8        94\t11\t00\t55\tFF\tFF\tFF\t1F\r\n       645  0CF104A7   00000004    8        F0\t60\t22\tFC\tFF\tFF\tFF\t3E\r\n       644  0CF103A7   00000004    8        17\t1F\t08\t60\tB1\t1F\t08\t3E\r\n       644  0C3C4D4A   00000004    8        BE\tFF\tFF\t7F\t18\tFF\tFF\t3E\r\n       643  0CF102A7   00000004    8        30\t75\tE0\t2E\t80\tFF\tFF\tFD\r\n       643  0CF101A7   00000004    8        68\t00\t97\tCC\t00\t15\t39\t3A\r\n       642  18F11FF0   00000004    8        FF\t3F\t90\t68\t88\t1B\t10\tEC\r\n       632  1FFFFFFF   00000004    8        00\t20\tFF\tFF\tFF\tFF\tFF\tFF\r\n       623  0CF102A7   00000004    8        30\t75\tE0\t2E\t80\tFF\tFF\tFD\r\n       623  0CF101A7   00000004    8        68\t00\t97\tCC\t00\t15\t39\t39\r\n       647  18F108A7   00000004    8        F0\t00\t00\tFF\tFF\tFF\tFF\t3F\r\n       646  18F106A7   00000004    8        00\tF7\tFF\tFF\tFF\tFF\tFF\t7D\r\n       645  0CF105A7   00000004    8        94\t11\t00\t55\tFF\tFF\tFF\t1F\r\n       645  0CF104A7   00000004    8        F0\t60\t22\tFC\tFF\tFF\tFF\t3E\r\n       644  0CF103A7   00000004    8        17\t1F\t08\t60\tB1\t1F\t08\t3E\r\n       644  0C3C4D4A   00000004    8        BE\tFF\tFF\t7F\t18\tFF\tFF\t3E\r\n       643  0CF102A7   00000004    8        30\t75\tE0\t2E\t80\tFF\tFF\tFD\r\n       643  0CF101A7   00000004    8        68\t00\t97\tCC\t00\t15\t39\t3A\r\n       642  18F11FF0   00000004    8        FF\t3F\t90\t68\t88\t1B\t10\tEC\r\n       632  1FFFFFFF   00000004    8        00\t20\tFF\tFF\tFF\tFF\tFF\tFF\r\n       623  0CF102A7   00000004    8        30\t75\tE0\t2E\t80\tFF\tFF\tFD\r\n       647  18F120F0   00000004    8        2B\t75\t60\tB1\tB0\t01\tFF\tFF\r\n       647  18F108A7   00000004    8        F0\t00\t00\tFF\tFF\tFF\tFF\t3F\r\n       646  18F106A7   00000004    8        00\tF7\tFF\tFF\tFF\tFF\tFF\t7D\r\n       645  0CF105A7   00000004    8        94\t11\t00\t55\tFF\tFF\tFF\t1F\r\n       645  0CF104A7   00000004    8        F0\t60\t22\tFC\tFF\tFF\tFF\t3E\r\n       644  0CF103A7   00000004    8        17\t1F\t08\t60\tB1\t1F\t08\t3E\r\n       644  0C3C4D4A   00000004    8        BE\tFF\tFF\t7F\t18\tFF\tFF\t3E\r\n       643  0CF102A7   00000004    8        30\t75\tE0\t2E\t80\tFF\tFF\tFD\r\n       643  0CF101A7   00000004    8        68\t00\t97\tCC\t00\t15\t39\t3A\r\n       642  18F11FF0   00000004    8        FF\t3F\t90\t68\t88\t1B\t10\tEC\r\n       632  1FFFFFFF   00000004    8        00\t20\tFF\tFF\tFF\tFF\tFF\tFF\r\n       648  18F121F0   00000004    8        09\t16\t00\t00\tFF\tFF\tB0\t01\r\n       647  18F120F0   00000004    8        2B\t75\t60\tB1\tB0\t01\tFF\tFF\r\n       647  18F108A7   00000004    8        F0\t00\t00\tFF\tFF\tFF\tFF\t3F\r\n       646  18F106A7   00000004    8        00\tF7\tFF\tFF\tFF\tFF\tFF\t7D\r\n       645  0CF105A7   00000004    8        94\t11\t00\t55\tFF\tFF\tFF\t1F\r\n       645  0CF104A7   00000004    8        F0\t60\t22\tFC\tFF\tFF\tFF\t3E\r\n       644  0CF103A7   00000004    8        17\t1F\t08\t60\tB1\t1F\t08\t3E\r\n       644  0C3C4D4A   00000004    8        BE\tFF\tFF\t7F\t18\tFF\tFF\t3E\r\n       643  0CF102A7   00000004    8        30\t75\tE0\t2E\t80\tFF\tFF\tFD\r\n       643  0CF101A7   00000004    8        68\t00\t97\tCC\t00\t15\t39\t3A\r\n       642  18F11FF0   00000004    8        FF\t3F\t90\t68\t88\t1B\t10\tEC\r\n       648  18FB01A7   00000004    8        FF\t1F\tFF\tFF\tFF\tFF\tFF\tFF\r\n       648  18F121F0   00000004    8        09\t16\t00\t00\tFF\tFF\tB0\t01\r\n       647  18F120F0   00000004    8        2B\t75\t60\tB1\tB0\t01\tFF\tFF\r\n       647  18F108A7   00000004    8        F0\t00\t00\tFF\tFF\tFF\tFF\t3F\r\n       646  18F106A7   00000004    8        00\tF7\tFF\tFF\tFF\tFF\tFF\t7D\r\n       645  0CF105A7   00000004    8        94\t11\t00\t55\tFF\tFF\tFF\t1F\r\n       645  0CF104A7   00000004    8        F0\t60\t22\tFC\tFF\tFF\tFF\t3E\r\n       644  0CF103A7   00000004    8        17\t1F\t08\t60\tB1\t1F\t08\t3E\r\n       644  0C3C4D4A   00000004    8        BE\tFF\tFF\t7F\t18\tFF\tFF\t3E\r\n       643  0CF102A7   00000004    8        30\t75\tE0\t2E\t80\tFF\tFF\tFD\r\n       643  0CF101A7   00000004    8        68\t00\t97\tCC\t00\t15\t39\t3A\r\n       649  18FEF117   00000004    8        F7\t97\tCC\tCF\tFF\tFF\tFF\tFF\r\n       648  18FB01A7   00000004    8        FF\t1F\tFF\tFF\tFF\tFF\tFF\tFF\r\n       648  18F121F0   00000004    8        09\t16\t00\t00\tFF\tFF\tB0\t01\r\n       647  18F120F0   00000004    8        2B\t75\t60\tB1\tB0\t01\tFF\tFF\r\n       647  18F108A7   00000004    8        F0\t00\t00\tFF\tFF\tFF\tFF\t3F\r\n       646  18F106A7   00000004    8        00\tF7\tFF\tFF\tFF\tFF\tFF\t7D\r\n       645  0CF105A7   00000004    8        94\t11\t00\t55\tFF\tFF\tFF\t1F\r\n       645  0CF104A7   00000004    8        F0\t60\t22\tFC\tFF\tFF\tFF\t3E\r\n       644  0CF103A7   00000004    8        17\t1F\t08\t60\tB1\t1F\t08\t3E\r\n       644  0C3C4D4A   00000004    8        BE\tFF\tFF\t7F\t18\tFF\tFF\t3E\r\n       643  0CF102A7   00000004    8        30\t75\tE0\t2E\t80\tFF\tFF\tFD\r\n       649  1FFFFFFF   00000004    8        00\t20\tFF\tFF\tFF\tFF\tFF\tFF\r\n       649  18FEF117   00000004    8        F7\t97\tCC\tCF\tFF\tFF\tFF\tFF\r\n       648  18FB01A7   00000004    8        FF\t1F\tFF\tFF\tFF\tFF\tFF\tFF\r\n       648  18F121F0   00000004    8        09\t16\t00\t00\tFF\tFF\tB0\t01\r\n       647  18F120F0   00000004    8        2B\t75\t60\tB1\tB0\t01\tFF\tFF\r
